vi "Move Control To ConPane.vi"(4 "Pane":refnum<vi>, 6 "Ref. VI":refnum<vi>, 8 "error in":errorcluster, 9 "Conpane Map":T1(c390), 10 "Terminal Index":i32) -> (0 "error out":errorcluster, 2 "Control":refnum<vi>)   [LabVIEW 2021, in "_Msg Rescript.lvlib" / "_Msg Rescript.lvclass"]
uses:
  _Msg Rescript.lvclass
  <vilib>/Utility/miscctls.llb/LVPositionTypeDef.ctl
  _Msg Rescript.lvclass/_Msg Rescript.ctl
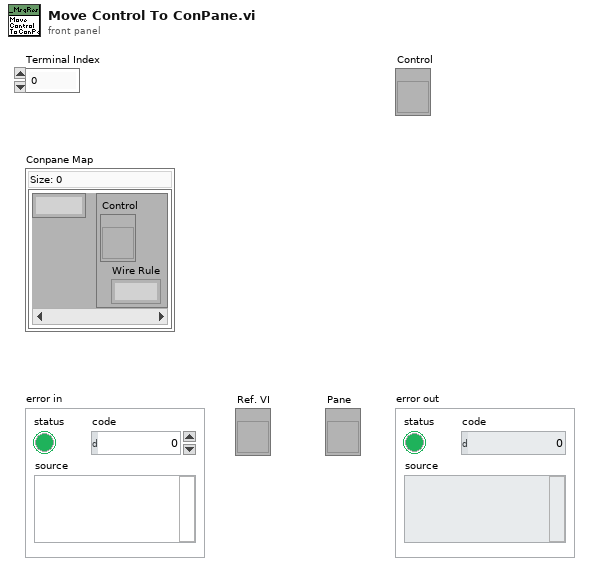
[diagram p1: front panel]
types:
  T1 = map{i32, cluster{"Control":refnum<vi>, "Wire Rule":enum16{"Invalid Wire Rule", "Required", "Recommended", "Optional", "Dynamic Dispatch"}}}
  T2 = typedef "LVPositionTypeDef.ctl" = cluster{"Left":i32, "Top":i32}
  T3 = cluster{"Control":refnum<vi>, "Wire Rule":enum16{"Invalid Wire Rule", "Required", "Recommended", "Optional", "Dynamic Dispatch"}}
  T4 = enum16{"Invalid Wire Rule", "Required", "Recommended", "Optional", "Dynamic Dispatch"}
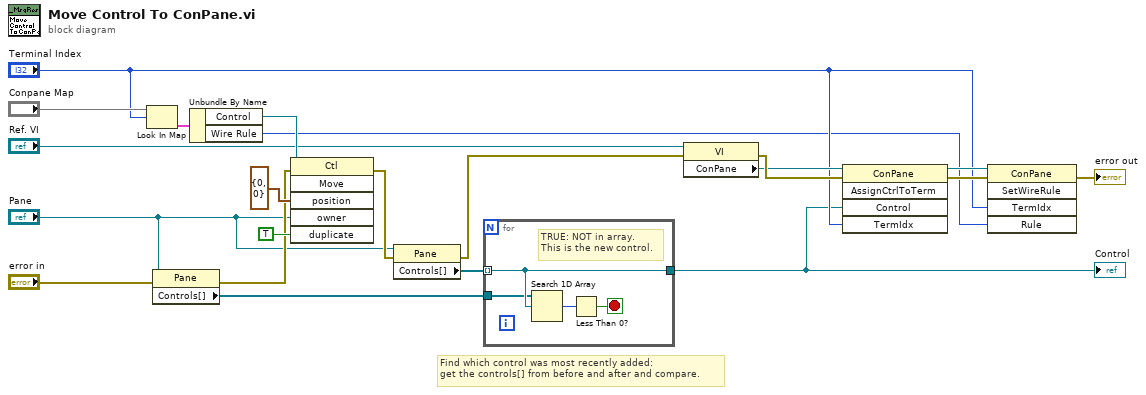
[diagram p0: block diagram]
diagram:
  # "Find which control was most recently added:\nget the controls[] from before and after and compare."
  n1 = Look In Map(map="Conpane Map", key="Terminal Index") -> (value=w21:T3)  [unwired: 1 in, 1 out]
  n2 = property class="Pane"(reference="Pane", error in="error in") -> (error out=w13:errorcluster, "Controls[]"=w11:refnum<vi>[])  [unwired: 1 out]
  n3 = Unbundle By Name(w21) -> ("Control"=w17:refnum<vi>, "Wire Rule"=w1:T4)
  n4 = invoke class="Ctl" method="Move"(reference=w17, error in=w13, "position"=T2 {"Left"=0, "Top"=0}, "owner"="Pane", "duplicate"=TRUE ("Duplicate? (F)")) -> (error out=w10:errorcluster)  [unwired: 1 in, 5 out]
  n5 = property class="Pane"(reference="Pane", error in=w10) -> (error out=w9:errorcluster, "Controls[]"=w12:refnum<vi>[])  [unwired: 1 out]
  n6 = for {
    tunnel: w12 -> [w25] mode=indexing
    tunnel: w11 -> [w24]
    tunnel: [w25] -> w2
    stop <- w22 stop-if-true
    # "TRUE: NOT in array.\nThis is the new control."
    n7 = Search 1D Array(1D array=w24, element=w25) -> (index of element=w23:i32)  [unwired: 1 in]
    n8 = Less Than 0?(x=w23) -> (x < 0?=w22:bool)
  }
  "Control" <- w2
  n9 = property class="VI"(reference="Ref. VI", error in=w9) -> (error out=w16:errorcluster, "ConPane"=w14:refnum<vi>)  [unwired: 1 out]
  n10 = invoke class="ConPane" method="AssignCtrlToTerm"(reference=w14, error in=w16, "Control"=w2, "TermIdx"="Terminal Index") -> (reference out=w18:refnum<vi>, error out=w15:errorcluster)  [unwired: 1 in, 3 out]
  n11 = invoke class="ConPane" method="SetWireRule"(reference=w18, error in=w15, "TermIdx"="Terminal Index", "Rule"=w1) -> (error out=→"error out":errorcluster)  [unwired: 1 in, 4 out]
